vi "RSZVL Sample Code.vi"() -> ()   [LabVIEW 2015]
panel:
  in  "File Name (\"D:\\user\\data\")":string="Band A RX" caption="Recall Cal"
  in  "Error Correction":bool
  out "Trace Freq":dbl[](array[numeric])
  out "XY Graph":cluster{dbl[], "Trace Data":dbl[]}(graph)
  out "Step Size":dbl format="%^.3e"
  out "Number Of Points":i32
  in  "Number Of Points (201)":i32=201
  in  "Source Power (-10.0)":dbl=-10.0 format="%^.3e"
  in  "Stop Frequency (3.0e+9)":dbl=3000000000.0 format="%^.3e"
  in  "Start Frequency (0.0)":dbl format="%^.3e"
  in  "Trace Name (\"Trc1\")":string="Trc1"
  out "Trace Data":dbl[](array[numeric]) format="%^.3e"
  in  "Acquire":bool
  out "error out":errorcluster
  in  "stop":bool
  in  "VISA resource name":refnum<visa-resource-name>="RSZVL"
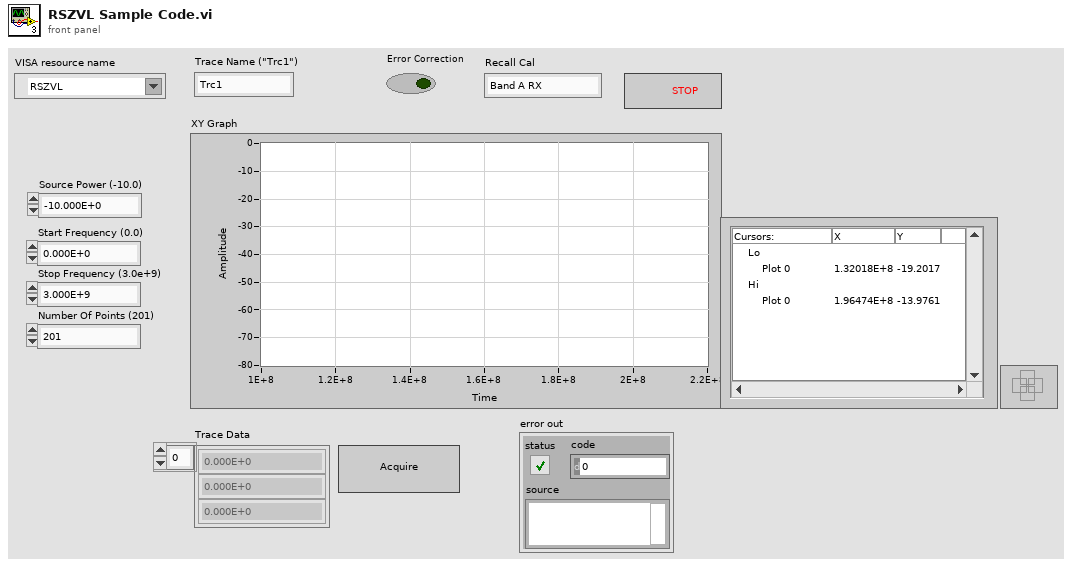
[diagram p1: front panel]
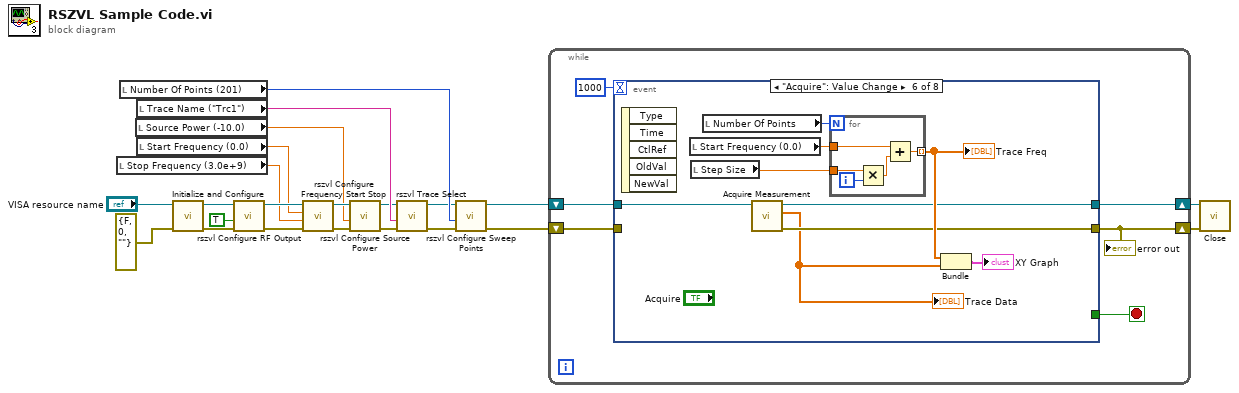
[diagram p0: block diagram]
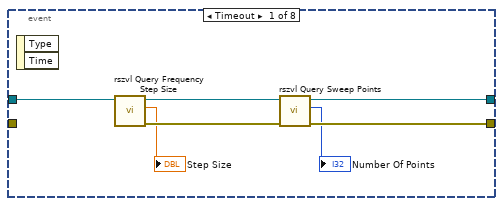
[diagram p2: hidden frame]
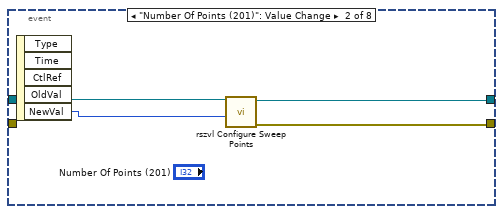
[diagram p3: hidden frame]
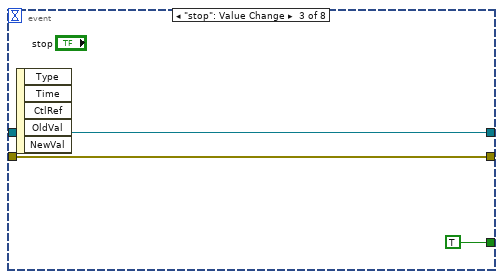
[diagram p4: hidden frame]
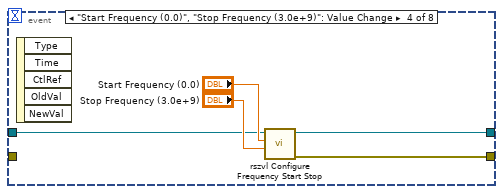
[diagram p5: hidden frame]
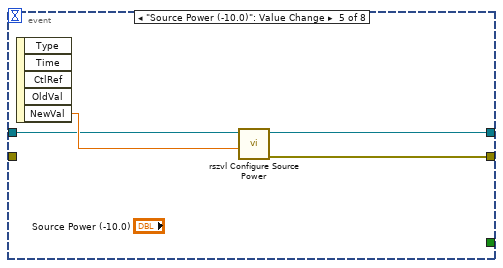
[diagram p6: hidden frame]
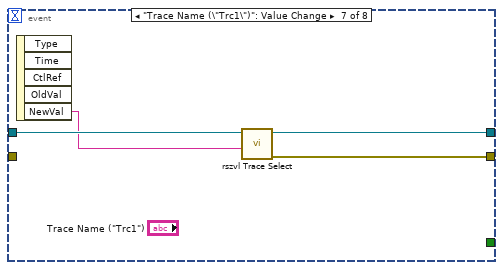
[diagram p7: hidden frame]
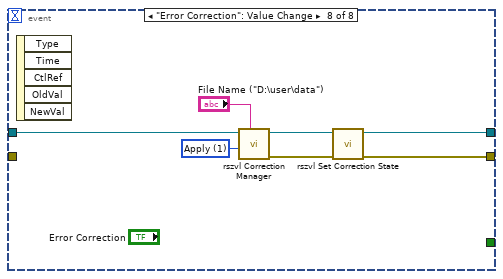
[diagram p8: hidden frame]
diagram:
  n1 = local read "Stop Frequency (3.0e+9)"() -> (w14:dbl)
  n2 = local read "Number Of Points (201)"() -> (w7:i32)
  n3 = local read "Source Power (-10.0)"() -> (w11:dbl)
  n4 = local read "Trace Name (\"Trc1\")"() -> (w10:string)
  n5 = local read "Start Frequency (0.0)"() -> (w15:dbl)
  n6 = call "Initialize and Configure.vi"("error in (no error)"=errorcluster {"status"=FALSE, "code"=0, "source"=""}, "VISA resource name"="VISA resource name") -> ("error out"=w20:errorcluster, "VISA resource name out"=w19:refnum<visa-resource-name>)  [unwired: 8 in]
  n7 = call <instrlib>:"rszvl Configure RF Output.vi"("error in (no error)"=w20, "RF Output (On)"=TRUE, "VISA resource name"=w19) -> ("error out"=w16:errorcluster, "VISA resource name out"=w17:refnum<visa-resource-name>)  [unwired: 7 in]
  n8 = call <instrlib>:"rszvl Configure Frequency Start Stop.vi"("error in (no error)"=w16, "Stop Frequency (3.0e+9)"=w14, "Start Frequency (0.0)"=w15, "VISA resource name"=w17) -> ("error out"=w12:errorcluster, "VISA resource name out"=w13:refnum<visa-resource-name>)  [unwired: 6 in]
  n9 = call <instrlib>:"rszvl Configure Source Power.vi"("error in (no error)"=w12, "Source Power (-10.0)"=w11, "VISA resource name"=w13) -> ("error out"=w8:errorcluster, "VISA resource name out"=w9:refnum<visa-resource-name>)  [unwired: 7 in]
  n10 = call <instrlib>:"rszvl Trace Select.vi"("error in (no error)"=w8, "Trace Name (\"Trc1\")"=w10, "VISA resource name"=w9) -> ("error out"=w4:errorcluster, "VISA resource name out"=w6:refnum<visa-resource-name>)  [unwired: 7 in]
  n11 = call <instrlib>:"rszvl Configure Sweep Points.vi"("error in (no error)"=w4, "Number Of Points (201)"=w7, "VISA resource name"=w6) -> ("error out"=w3:errorcluster, "VISA resource name out"=w5:refnum<visa-resource-name>)  [unwired: 7 in]
  n12 = while {
    shift-right: [w25] -> w2
    shift-left: w3 -> [w27]
    shift-right: [w26] -> w1
    shift-left: w5 -> [w28]
    stop <- w24 stop-if-true
    n13 = event shown="[5] \"Acquire\": Value Change" {
      selector: _ -> [_ _ _ _ _ _ _ _]
      dyn-events: _ -> [_ _ _ _ _ _ _ _]
      timeout: 1000 -> [_ _ _ _ _ _ _ _]
      tunnel: w28 -> [w35 w39 w42 w45 w49 w52 w68 w71]
      tunnel: w27 -> [_ _ w41 _ _ _ _ _]
      tunnel: [w31 w38 w42 w44 w48 w55 w66 w72] -> w26
      tunnel: [w32 w37 w41 w43 w51 w54 w69 w73] -> w25
      tunnel: [_ _ TRUE _ _ _ _ _] -> w24
      event Timeout {
        n14 = event-data() -> ()  [unwired: 1 in, 2 out]
        n15 = call <instrlib>:"rszvl Query Frequency Step Size.vi"("VISA resource name"=w35) -> ("error out"=w33:errorcluster, "Step Size"=→"Step Size":dbl, "VISA resource name out"=w34:refnum<visa-resource-name>)  [unwired: 8 in]
        n16 = call <instrlib>:"rszvl Query Sweep Points.vi"("error in (no error)"=w33, "VISA resource name"=w34) -> ("error out"=w32:errorcluster, "Number Of Points"=→"Number Of Points":i32, "VISA resource name out"=w31:refnum<visa-resource-name>)  [unwired: 7 in]
      }
      event "Number Of Points (201)": Value Change {
        n17 = event-data() -> ("NewVal"=w36:i32)  [unwired: 1 in, 4 out]
        n18 = call <instrlib>:"rszvl Configure Sweep Points.vi"("Number Of Points (201)"=w36, "VISA resource name"=w39) -> ("error out"=w37:errorcluster, "VISA resource name out"=w38:refnum<visa-resource-name>)  [unwired: 8 in]
      }
      event "stop": Value Change {
        n19 = event-data() -> ()  [unwired: 1 in, 5 out]
      }
      event "Start Frequency (0.0)", "Stop Frequency (3.0e+9)": Value Change {
        n20 = event-data() -> ()  [unwired: 1 in, 5 out]
        n21 = call <instrlib>:"rszvl Configure Frequency Start Stop.vi"("Stop Frequency (3.0e+9)"="Stop Frequency (3.0e+9)", "Start Frequency (0.0)"="Start Frequency (0.0)", "VISA resource name"=w45) -> ("error out"=w43:errorcluster, "VISA resource name out"=w44:refnum<visa-resource-name>)  [unwired: 7 in]
      }
      event "Source Power (-10.0)": Value Change {
        n22 = event-data() -> ("NewVal"=w50:dbl)  [unwired: 1 in, 4 out]
        n23 = call <instrlib>:"rszvl Configure Source Power.vi"("Source Power (-10.0)"=w50, "VISA resource name"=w49) -> ("error out"=w51:errorcluster, "VISA resource name out"=w48:refnum<visa-resource-name>)  [unwired: 8 in]
      }
      event "Acquire": Value Change {
        n24 = event-data() -> ()  [unwired: 1 in, 5 out]
        n25 = local read "Start Frequency (0.0)"() -> (w60:dbl)
        n26 = local read "Step Size"() -> (w59:dbl)
        n27 = local read "Number Of Points"() -> (w58:i32)
        n28 = call "Acquire Measurement.vi"("VISA resource name"=w52) -> ("error out"=w54:errorcluster, "Trace Data"=w53:dbl[], "VISA resource name out"=w55:refnum<visa-resource-name>)  [unwired: 8 in]
        "Trace Data" <- w53
        n29 = for {
          N: w58 -> [_]
          tunnel: w59 -> [w65]
          tunnel: w60 -> [w62]
          tunnel: [w61] -> w57 mode=indexing
          i -> [w64]
          n30 = Multiply(x=w65, y=w64) -> (x*y=w63:dbl)
          n31 = Add(x=w62, y=w63) -> (x+y=w61:dbl)
        }
        "Trace Freq" <- w57
        n32 = Bundle(w57, "Trace Data"=w53) -> (→"XY Graph":cluster{dbl[], "Trace Data":dbl[]})  [unwired: 1 in]
      }
      event "Trace Name (\"Trc1\")": Value Change {
        n33 = event-data() -> ("NewVal"=w67:string)  [unwired: 1 in, 4 out]
        n34 = call <instrlib>:"rszvl Trace Select.vi"("Trace Name (\"Trc1\")"=w67, "VISA resource name"=w68) -> ("error out"=w69:errorcluster, "VISA resource name out"=w66:refnum<visa-resource-name>)  [unwired: 8 in]
      }
      event "Error Correction": Value Change {
        w70 = 1 items=["Copy", "Apply", "Resolve Pool Link", "Delete"] ("Operation to be Performed (Copy)")
        n35 = event-data() -> ()  [unwired: 1 in, 5 out]
        n36 = call <instrlib>:"rszvl Correction Manager.vi"("File Name (\"D:\\user\\data\")"="File Name (\"D:\\user\\data\")", "Operation to be Performed (Copy)"=w70, "VISA resource name"=w71) -> ("error out"=w74:errorcluster, "VISA resource name out"=w75:refnum<visa-resource-name>)  [unwired: 7 in]
        n37 = call <instrlib>:"rszvl Set Correction State.vi"("error in (no error)"=w74, "VISA resource name"=w75) -> ("error out"=w73:errorcluster, "VISA resource name out"=w72:refnum<visa-resource-name>)  [unwired: 8 in]
      }
    }
    "error out" <- w25
  }
  n38 = call "Close.vi"("error in (no error)"=w2, "VISA resource name"=w1) -> ()  [unwired: 9 in, 1 out]
